vi "pthread_barrier_init.vi"(8 "error in (no error)":errorcluster, 9 "count":u32, 10 "barrier attr ptr in":u64, 11 "barrier ptr in":u64) -> (0 "error out":errorcluster, 2 "barrier attr ptr out":u64, 3 "barrier ptr out":u64)   [LabVIEW 2013, in "POSIX Threads.lvlib" / "POSIX Thread Object.lvclass"]
uses:
  POSIX Thread Object.lvclass
  Controls/pthread functions.ctl
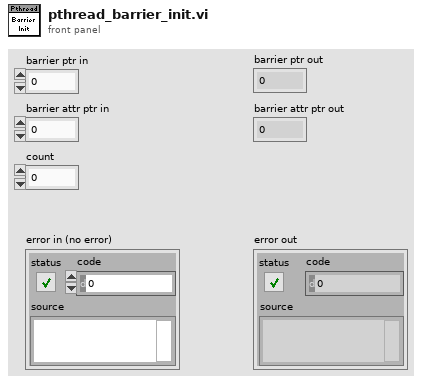
[diagram p1: front panel]
types:
  T1 = typedef "POSIX Threads.lvlib/POSIX Thread Object.lvclass/pthread functions.ctl" = enum16{"unspecified", "pthread_condattr_init", "pthread_condattr_destroy", "pthread_condattr_getclock", "pthread_condattr_setclock", "pthread_condattr_getpshared", "pthread_condattr_setpshared", "pthread_cond_init", "pthread_cond_destroy", "pthread_cond_broadcast", "pthread_cond_signal", "pthread_cond_timedwait", "pthread_cond_wait", "pthread_mutexattr_init", "pthread_mutexattr_destroy", "pthread_mutexattr_getprioceiling", "pthread_mutexattr_setprioceiling", "pthread_mutexattr_getprotocol", "pthread_mutexattr_setprotocol", "pthread_mutexattr_getpshared", "pthread_mutexattr_setpshared", "pthread_mutexattr_gettype", "pthread_mutexattr_settype", "pthread_mutex_init", "pthread_mutex_destroy", "pthread_mutex_getprioceiling", "pthread_mutex_setprioceiling", "pthread_mutex_lock", "pthread_mutex_timedlock", "pthread_mutex_trylock", "pthread_mutex_unlock", "sem_destroy", "sem_getvalue", "sem_init", "sem_post", "sem_timedwait", "sem_trywait", "sem_wait", "barrier_init", "barrier_destroy", "barrier_wait", "barrierattr_init", "barrierattr_destroy", "barrierattr_getpshared", "barrierattr_setpshared"}
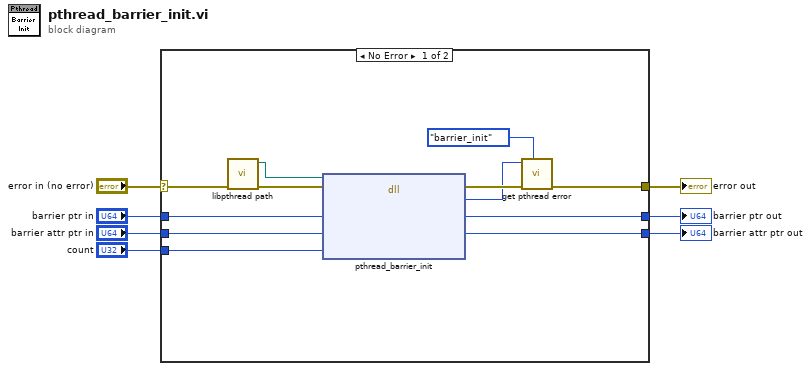
[diagram p0: block diagram]
diagram:
  n1 = case shown="No Error" "error in (no error)" {
    selector: "error in (no error)" -> [w19 w22]
    tunnel: "barrier ptr in" -> [w18 w21]
    tunnel: [w17 w22] -> w5
    tunnel: [w16 w21] -> w4
    tunnel: "barrier attr ptr in" -> [w15 w20]
    tunnel: [w14 w20] -> w2
    tunnel: "count" -> [w8 _]
    frame No Error {
      n2 = call "libpthread path.vi"("error in (no error)"=w19) -> ("error out"=w12:errorcluster, "path to libpthread"=w13:path)  [unwired: 9 in]
      n3 = dll-call lib="?" fn="pthread_barrier_init"(path in=w13, error in=w12, "barrier"=w18, "barrier attr"=w15, "count"=w8) -> (error out=w11:errorcluster, "errno"=w10:i32, "barrier"=w16:u64, "barrier attr"=w14:u64)  [unwired: 2 in, 1 out]
      n4 = call "get pthread error.vi"("function"=pthread_functions."barrier_init", "error in (no error)"=w11, "errno"=w10) -> ("error out"=w17:errorcluster)  [unwired: 8 in]
    }
    frame Error {
    }
  }
  "error out" <- w5
  "barrier ptr out" <- w4
  "barrier attr ptr out" <- w2
